vi "Read Instrument Names.vi"(8 "error in (no error)":errorcluster, 10 "Instrument Classes":T1) -> (0 "error out":errorcluster, 2 "Array":string[](array[string]))   [LabVIEW 2019, in "Control Experiment.lvclass"]
uses:
  Control Experiment.lvclass
  <userlib>/LevyLab/Instrument Framework/Instrument/Instrument.lvclass
  C:/Program Files/National Instruments/LabVIEW 2019/vi.lib/JKI/JKI SMO/SMO/SMO.lvclass
  <userlib>/LevyLab/Instrument Framework/Instrument Types/Amplifier/Instrument.Amplifier.lvclass
  <userlib>/LevyLab/Instrument Framework/Instrument Types/Lockin/Instrument.LockinAPI.lvclass
  <userlib>/LevyLab/Instrument Framework/Instrument Types/Cryostat/Instrument.Cryostat.lvclass
  <userlib>/LevyLab/Instrument Framework/Instrument Types/CBridge/Instrument.CBridge.lvclass
  <userlib>/LevyLab/Instrument Framework/Instrument Types/Delay Line/Instrument.DelayLine.lvclass
  <userlib>/LevyLab/Instrument Framework/Instrument Types/Strain/Instrument.Strain.lvclass
  <userlib>/LevyLab/Instrument Framework/Instrument Types/VNA/Instrument.VNA.lvclass
  <userlib>/LevyLab/Instrument Framework/Instrument Types/VSource/Instrument.VSource.lvclass
  Typedefs/Instrument Classes--cluster.ctl
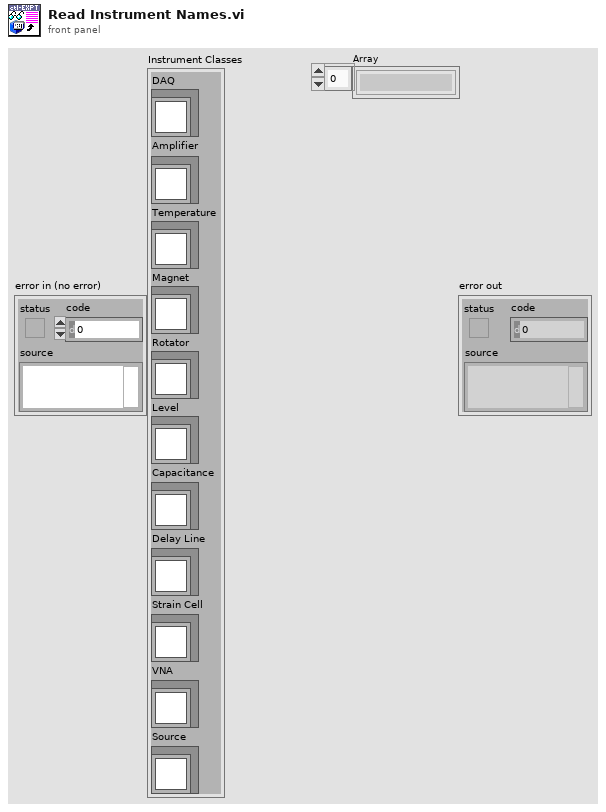
[diagram p1: front panel]
types:
  T1 = typedef "Control Experiment.lvclass/Instrument Classes--cluster.ctl" = cluster{"DAQ":refnum<class "Instrument.LockinAPI.lvclass">, "Amplifier":refnum<class "Instrument.Amplifier.lvclass">, "Temperature":refnum<class "Instrument.Cryostat.lvclass">, "Magnet":refnum<class "Instrument.Cryostat.lvclass">, "Rotator":refnum<class "Instrument.Cryostat.lvclass">, "Level":refnum<class "Instrument.Cryostat.lvclass">, "Capacitance":refnum<class "Instrument.CBridge.lvclass">, "Delay Line":refnum<class "Instrument.DelayLine.lvclass">, "Strain Cell":refnum<class "Instrument.Strain.lvclass">, "VNA":refnum<class "Instrument.VNA.lvclass">, "Source":refnum<class "Instrument.VSource.lvclass">}
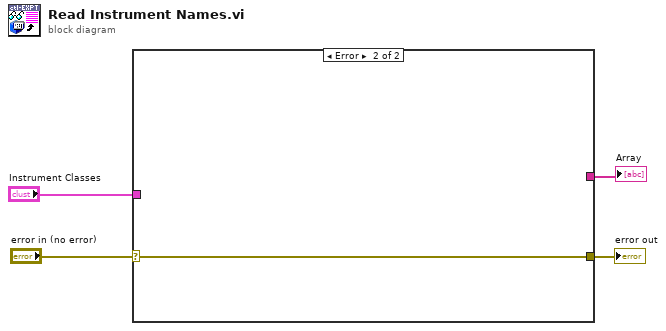
[diagram p0: block diagram]
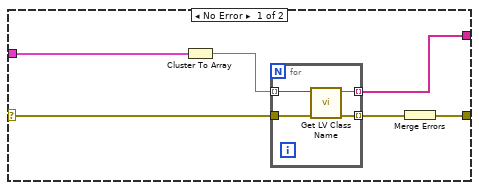
[diagram p2: hidden frame]
diagram:
  n1 = case shown="Error" "error in (no error)" {
    selector: "error in (no error)" -> [w10 w15]
    tunnel: [w7 _] -> w3
    tunnel: [w8 w15] -> w2
    tunnel: "Instrument Classes" -> [w5 _]
    frame No Error {
      n2 = Cluster To Array(cluster=w5) -> (array=w6:refnum<class "Instrument.lvclass">[])
      n3 = for {
        tunnel: w6 -> [w11] mode=indexing
        tunnel: w10 -> [w14]
        tunnel: [w13] -> w9 mode=indexing
        tunnel: [w12] -> w7 mode=indexing
        n4 = call <vilib>:"Get LV Class Name.vi"("error in (no error)"=w14, "object"=w11) -> ("error out"=w13:errorcluster, "class name"=w12:string)  [unwired: 8 in]
      }
      n5 = Merge Errors(w9) -> (w8:errorcluster)
    }
    frame Error {
    }
  }
  "error out" <- w2
  "Array" <- w3
